vi "ReadFromMultiFile.vi"(8 "error in (no error)":errorcluster, 10 "FilePathArray":path[](array[path]), 11 "RawData":T2(array[cluster])) -> (0 "error out":errorcluster, 2 "MultiPlot":T1, 3 "RawDataOut":T2(array[cluster]))   [LabVIEW 2012]
doc: "读取多个文件，一共有6种波形，分别保存数据到各自的数组里面。\nname: 蒋松\nEmail：jiangsong@outlook.com"
uses:
  <vilib>/Utility/file.llb/Read From Spreadsheet File (DBL).vi
panel:
  # "VI INPUTS"
  # "VI OUTPUTS"
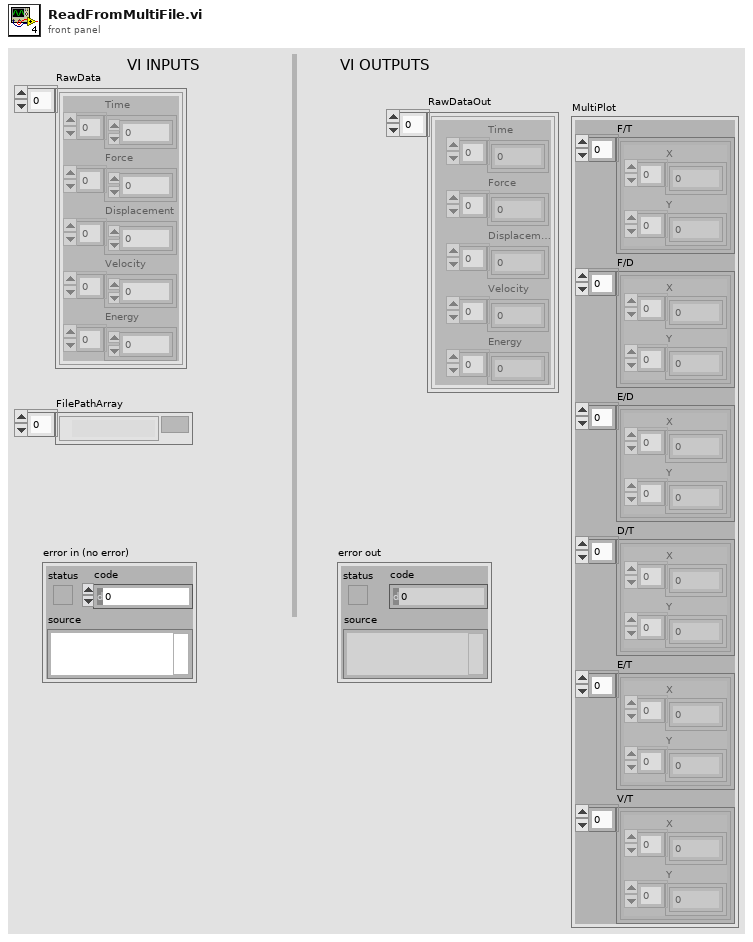
[diagram p1: front panel]
types:
  T1 = cluster{"F/T":cluster{"X":dbl[], "Y":dbl[]}[], "F/D":cluster{"X":dbl[], "Y":dbl[]}[], "E/D":cluster{"X":dbl[], "Y":dbl[]}[], "D/T":cluster{"X":dbl[], "Y":dbl[]}[], "E/T":cluster{"X":dbl[], "Y":dbl[]}[], "V/T":cluster{"X":dbl[], "Y":dbl[]}[]}
  T2 = cluster{"Time":dbl[], "Force":dbl[], "Displacement":dbl[], "Velocity":dbl[], "Energy":dbl[]}[]
  T3 = cluster{"Time":dbl[], "Force":dbl[], "Displacement":dbl[], "Velocity":dbl[], "Energy":dbl[]}
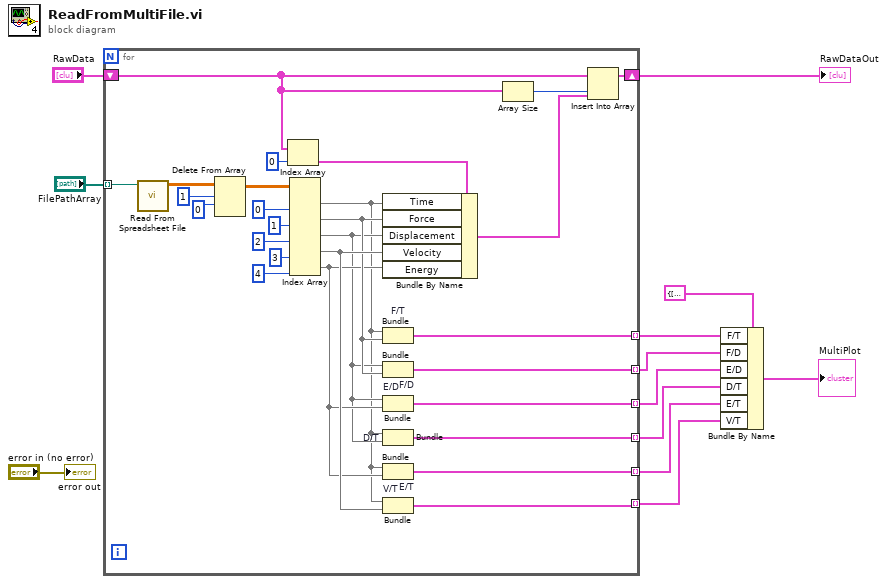
[diagram p0: block diagram]
diagram:
  n1 = for {
    tunnel: "FilePathArray" -> [w19] mode=indexing
    shift-right: [w38] -> w11
    shift-left: "RawData" -> [w39]
    tunnel: [w18] -> w6 mode=indexing
    tunnel: [w17] -> w5 mode=indexing
    tunnel: [w16] -> w4 mode=indexing
    tunnel: [w15] -> w3 mode=indexing
    tunnel: [w14] -> w2 mode=indexing
    tunnel: [w13] -> w1 mode=indexing
    n2 = call-poly <vilib>:"Read From Spreadsheet File.vi"("file path (dialog if empty)"=w19) -> ("all rows"=w35:dbl[][])  [unwired: 6 in, 4 out]
    n3 = Delete From Array(array=w35, length=1, index (row)=0) -> (array with subset deleted=w34:dbl[][])  [unwired: 1 in, 1 out]
    n4 = Index Array(array=w39, index=0) -> (element=w28:T3)
    n5 = Index Array(array=w34, index (col) #1=0 ("index (row)"), index (col) #2=1 ("index (row)"), index (col) #3=2 ("index (row)"), index (col) #4=3 ("index (row)"), index (col) #5=4 ("index (row)")) -> (element #1=w20:dbl[], element #2=w23:dbl[], element #3=w21:dbl[], element #4=w24:dbl[], element #5=w22:dbl[])  [unwired: 5 in]
    n6 = Bundle By Name(cluster=w28, "Time"=w20, "Force"=w23, "Displacement"=w21, "Velocity"=w24, "Energy"=w22) -> (w27:T3)
    n7 = Bundle "F/T"("all rows"=w20, "all rows"=w23) -> (w18:cluster{"all rows":dbl[], "all rows":dbl[]})  [unwired: 1 in]
    n8 = Bundle "F/D"("all rows"=w21, "all rows"=w23) -> (w17:cluster{"all rows":dbl[], "all rows":dbl[]})  [unwired: 1 in]
    n9 = Bundle "E/D"("all rows"=w21, "all rows"=w22) -> (w16:cluster{"all rows":dbl[], "all rows":dbl[]})  [unwired: 1 in]
    n10 = Bundle "D/T"("all rows"=w20, "all rows"=w21) -> (w15:cluster{"all rows":dbl[], "all rows":dbl[]})  [unwired: 1 in]
    n11 = Bundle "E/T"("all rows"=w20, "all rows"=w22) -> (w14:cluster{"all rows":dbl[], "all rows":dbl[]})  [unwired: 1 in]
    n12 = Bundle "V/T"("all rows"=w20, "all rows"=w24) -> (w13:cluster{"all rows":dbl[], "all rows":dbl[]})  [unwired: 1 in]
    n13 = Array Size(array=w39) -> (size(s)=w26:i32)
    n14 = Insert Into Array(array=w39, index=w26, new element=w27) -> (w38:T2)
  }
  "RawDataOut" <- w11
  n15 = Bundle By Name(cluster=T1 {"F/T"=[], "F/D"=[], "E/D"=[], "D/T"=[], "E/T"=[], "V/T"=[]} ("MultiPlot"), "F/T"=w6, "F/D"=w5, "E/D"=w4, "D/T"=w3, "E/T"=w2, "V/T"=w1) -> (→"MultiPlot":T1)
  "error out" <- "error in (no error)"
